vi "Union Rectangles.vi"(11 "Rectangles":T2(array[cluster])) -> (3 "Bounding Rect":T1)   [LabVIEW 2011]
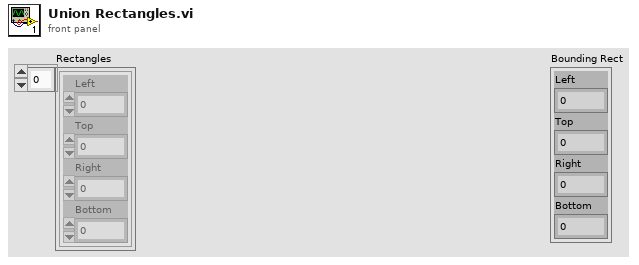
[diagram p1: front panel]
types:
  T1 = cluster{"Left":dbl, "Top":dbl, "Right":dbl, "Bottom":dbl}
  T2 = cluster{"Left":dbl, "Top":dbl, "Right":dbl, "Bottom":dbl}[]
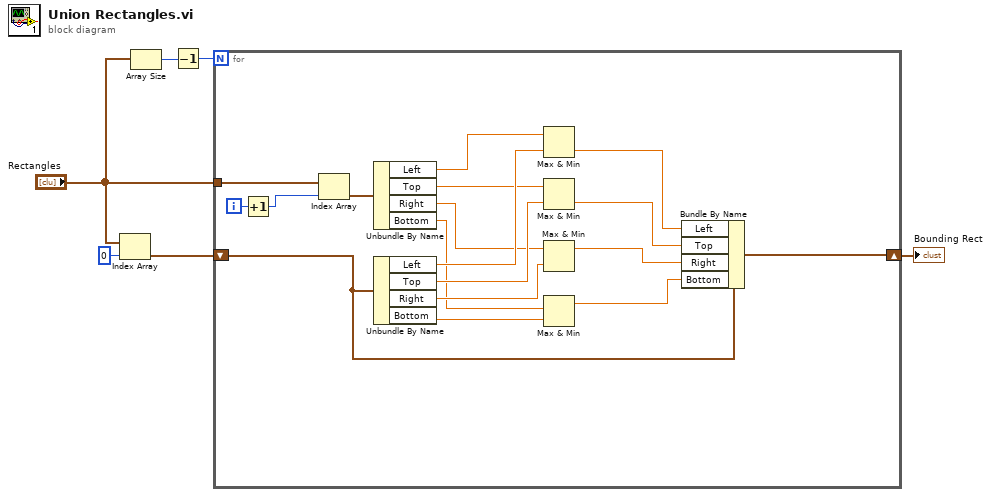
[diagram p0: block diagram]
diagram:
  n1 = Index Array(array="Rectangles", index=0) -> (element=w3:T1)
  n2 = Array Size(array="Rectangles") -> (size(s)=w6:i32)
  n3 = Decrement(x=w6) -> (x-1=w1:i32)
  n4 = for {
    N: w1 -> [_]
    tunnel: "Rectangles" -> [w23]
    shift-right: [w11] -> w2
    shift-left: w3 -> [w12]
    i -> [w24]
    n5 = Increment(x=w24) -> (x+1=w22:i32)
    n6 = Index Array(array=w23, index=w22) -> (element=w21:T1)
    n7 = Unbundle By Name(w21) -> ("Left"=w20:dbl, "Top"=w18:dbl, "Right"=w16:dbl, "Bottom"=w13:dbl)
    n8 = Unbundle By Name(w12) -> ("Left"=w19:dbl, "Top"=w17:dbl, "Right"=w15:dbl, "Bottom"=w14:dbl)
    n9 = Max & Min(x=w20, y=w19) -> (min(x,y)=w10:dbl)  [unwired: 1 out]
    n10 = Max & Min(x=w18, y=w17) -> (min(x,y)=w9:dbl)  [unwired: 1 out]
    n11 = Max & Min(x=w16, y=w15) -> (max(x,y)=w8:dbl)  [unwired: 1 out]
    n12 = Max & Min(x=w13, y=w14) -> (max(x,y)=w7:dbl)  [unwired: 1 out]
    n13 = Bundle By Name(cluster=w12, "Left"=w10, "Top"=w9, "Right"=w8, "Bottom"=w7) -> (w11:T1)
  }
  "Bounding Rect" <- w2
